vi "ObjectFabric ProductID2Object.vi"(1 "DG_Product":i32) -> (0 "BME_DG_Base":refnum<class "BME_DG_Base.lvclass">)   [LabVIEW 2009, in "POLARIS BME DG.lvlib" / "BME_DG_System.lvclass"]
uses:
  BME_DG_System.lvclass
  BME_DG_Base/BME_DG_Base.lvclass
  BME_DG_G08/BME_DG_G08.lvclass
  BME_DG_G02/BME_DG_G02.lvclass
  BME_DG_G05P2/BME_DG_G05P2.lvclass
  BME_DG_G05/BME_DG_G05.lvclass
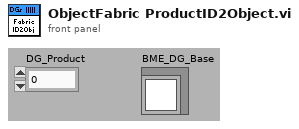
[diagram p1: front panel]
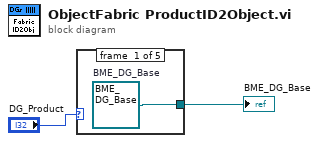
[diagram p0: block diagram]
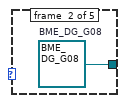
[diagram p2: hidden frame]
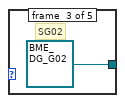
[diagram p3: hidden frame]
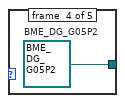
[diagram p4: hidden frame]
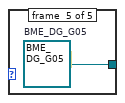
[diagram p5: hidden frame]
diagram:
  n1 = case shown="44, 45" "DG_Product" {
    tunnel: [w3 w4 refnum<class "BME_DG_G02.lvclass"> refnum ("BME_DG_G02.lvclass") w6 w7] -> w1
    frame #0 {
      w3 = refnum<class "BME_DG_Base.lvclass"> refnum  # BME_DG_Base
    }
    frame #1 {
      w4 = refnum<class "BME_DG_G08.lvclass"> refnum  # BME_DG_G08
    }
    frame #2 {
      # "SG02"
    }
    frame #3 {
      w6 = refnum<class "BME_DG_G05P2.lvclass"> refnum  # BME_DG_G05P2
    }
    frame #4 {
      w7 = refnum<class "BME_DG_G05.lvclass"> refnum  # BME_DG_G05
      # "G05"
    }
  }
  "BME_DG_Base" <- w1
